vi "Read Serial Input Channel IO.vi"(0 "serial input channel io":T1, 2 "select corrected csi-2 data":bool) -> (4 "csi-2 data":u8[](array[numeric]), 6 "csi-2 status":T4, 10 "output valid":bool)   [LabVIEW 2020, in "GettingStarted_Acq_Tap_148X_FPGA.lvlib"]
uses:
  GettingStarted_Acq_Tap_148X_FPGA.lvlib
  Types/CSI-2 Status.ctl
  Types/Serial Input Channel IO.ctl
  Types/Serial Input Channel IO 32b.ctl
  Types/Serial Input Channel IO 64b.ctl
  <vilib>/rvi/eio/common/nirviEmuTemplateMethod_errors.vi
  <vilib>/eio/EIONode/EIONode.xnode
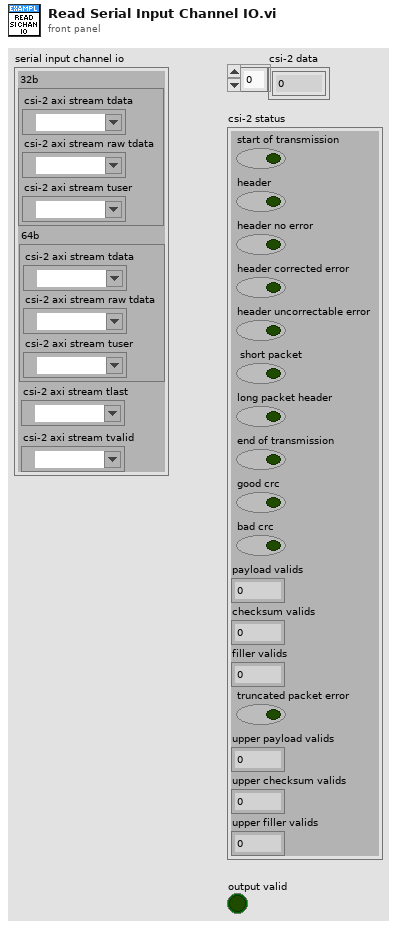
[diagram p1: front panel]
types:
  T1 = typedef "GettingStarted_Acq_Tap_148X_FPGA.lvlib/Serial Input Channel IO.ctl" = cluster{"32b":T2, "64b":T3, "csi-2 axi stream tlast":refnum<k21>, "csi-2 axi stream tvalid":refnum<k21>}
  T2 = typedef "GettingStarted_Acq_Tap_148X_FPGA.lvlib/Serial Input Channel IO 32b.ctl" = cluster{"csi-2 axi stream tdata":refnum<k21>, "csi-2 axi stream raw tdata":refnum<k21>, "csi-2 axi stream tuser":refnum<k21>}
  T3 = typedef "GettingStarted_Acq_Tap_148X_FPGA.lvlib/Serial Input Channel IO 64b.ctl" = cluster{"csi-2 axi stream tdata":refnum<k21>, "csi-2 axi stream raw tdata":refnum<k21>, "csi-2 axi stream tuser":refnum<k21>}
  T4 = typedef "GettingStarted_Acq_Tap_148X_FPGA.lvlib/CSI-2 Status.ctl" = cluster{"start of transmission":bool, "header":bool, "header no error":bool, "header corrected error":bool, "header uncorrectable error":bool, " short packet":bool, "long packet header":bool, "end of transmission":bool, "good crc":bool, "bad crc":bool, "payload valids":fxp<+,4,4>, "checksum valids":fxp<+,4,4>, "filler valids":fxp<+,4,4>, "truncated packet error":bool, "upper payload valids":fxp<+,4,4>, "upper checksum valids":fxp<+,4,4>, "upper filler valids":fxp<+,4,4>}
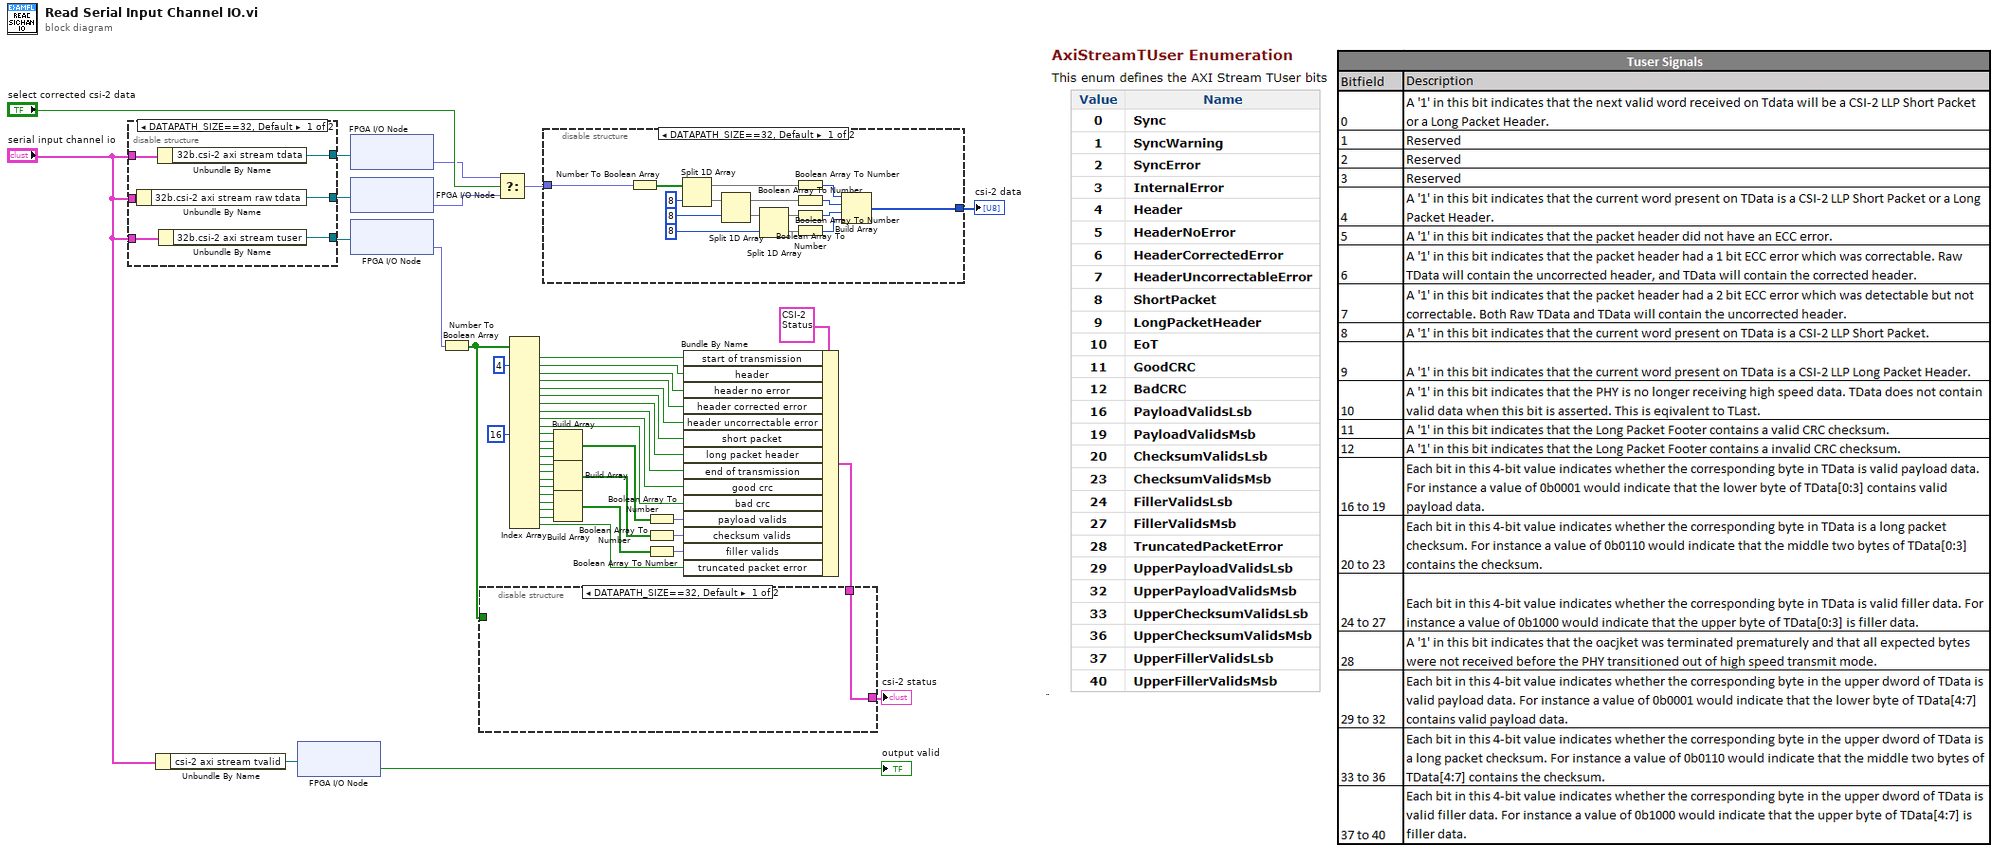
[diagram p0: block diagram]
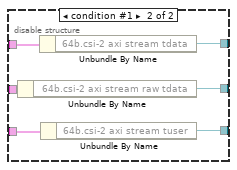
[diagram p2: hidden frame]
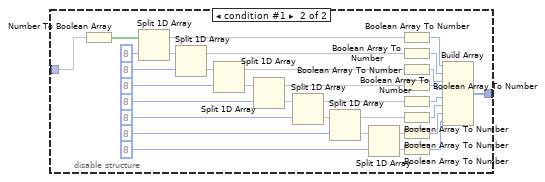
[diagram p3: hidden frame]
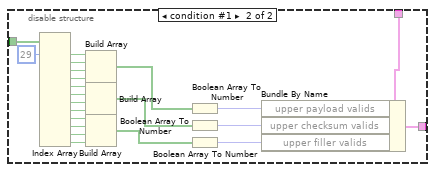
[diagram p4: hidden frame]
diagram:
  n1 = disable-structure shown="DATAPATH_SIZE==32, Default" {
    disable-tunnel: "serial input channel io" -> [w51 w59]
    disable-tunnel: "serial input channel io" -> [w52 w58]
    disable-tunnel: "serial input channel io" -> [w53 w57]
    disable-tunnel: [w50 w56] -> w6
    disable-tunnel: [w49 w55] -> w5
    disable-tunnel: [w48 w54] -> w4
    frame condition #0 (active) {
      n2 = Unbundle By Name(w52) -> ("32b.csi-2 axi stream raw tdata"=w49:refnum<k21>)
      n3 = Unbundle By Name(w53) -> ("32b.csi-2 axi stream tdata"=w48:refnum<k21>)
      n4 = Unbundle By Name(w51) -> ("32b.csi-2 axi stream tuser"=w50:refnum<k21>)
    }
    frame condition #1 {
      n5 = Unbundle By Name(w58) -> ("64b.csi-2 axi stream raw tdata"=w55:refnum<k21>)
      n6 = Unbundle By Name(w57) -> ("64b.csi-2 axi stream tdata"=w54:refnum<k21>)
      n7 = Unbundle By Name(w59) -> ("64b.csi-2 axi stream tuser"=w56:refnum<k21>)
    }
  }
  n8 = Unbundle By Name("serial input channel io") -> ("csi-2 axi stream tvalid"=w47:refnum<k21>)
  n9 = xnode "FPGA I/O Node"("FPGA I/O In"=w47) -> ("I/O Item"=→"output valid":bool)  [unwired: 1 out]
  n10 = xnode "FPGA I/O Node"("FPGA I/O In"=w4) -> ("I/O Item"=w42:fxp<+,32,32>)  [unwired: 1 out]
  n11 = xnode "FPGA I/O Node"("FPGA I/O In"=w5) -> ("I/O Item"=w41:fxp<+,32,32>)  [unwired: 1 out]
  n12 = xnode "FPGA I/O Node"("FPGA I/O In"=w6) -> ("I/O Item"=w45:fxp<+,32,32>)  [unwired: 1 out]
  n13 = Number To Boolean Array(number=w45) -> (Boolean array=w10:bool[])
  n14 = Select(t=w42, s="select corrected csi-2 data", f=w41) -> (s? t:f=w3:fxp<+,32,32>)
  n15 = Index Array(array=w10, index #2=4 ("index"), index #11=16 ("index")) -> (element #1=w46:bool, element #2=w38:bool, element #3=w37:bool, element #4=w36:bool, element #5=w35:bool, element #6=w34:bool, element #7=w33:bool, element #8=w32:bool, element #9=w31:bool, element #10=w30:bool, element #11=w28:bool, element #12=w27:bool, element #13=w26:bool, element #14=w25:bool, element #15=w23:bool, element #16=w22:bool, element #17=w21:bool, element #18=w20:bool, element #19=w17:bool, element #20=w16:bool, element #21=w15:bool, element #22=w14:bool, element #23=w1:bool)  [unwired: 21 in]
  n16 = disable-structure shown="DATAPATH_SIZE==32, Default" {
    disable-tunnel: w3 -> [w64 w94]
    disable-tunnel: [w60 w76] -> w2
    frame condition #0 (active) {
      n17 = Number To Boolean Array(number=w64) -> (Boolean array=w75:bool[])
      n18 = Split 1D Array(array=w75, index=8) -> (first subarray=w71:bool[], second subarray=w74:bool[])
      n19 = Split 1D Array(array=w74, index=8) -> (first subarray=w69:bool[], second subarray=w73:bool[])
      n20 = Split 1D Array(array=w73, index=8) -> (first subarray=w68:bool[], second subarray=w67:bool[])
      n21 = Boolean Array To Number(Boolean array=w71) -> (number=w72:u8)
      n22 = Boolean Array To Number(Boolean array=w69) -> (number=w70:u8)
      n23 = Boolean Array To Number(Boolean array=w68) -> (number=w66:u8)
      n24 = Boolean Array To Number(Boolean array=w67) -> (number=w65:u8)
      n25 = Build Array(w72, w70, w66, w65) -> (w60:u8[])
    }
    frame condition #1 {
      n26 = Number To Boolean Array(number=w94) -> (Boolean array=w107:bool[])
      n27 = Split 1D Array(array=w107, index=8) -> (first subarray=w103:bool[], second subarray=w106:bool[])
      n28 = Split 1D Array(array=w106, index=8) -> (first subarray=w101:bool[], second subarray=w105:bool[])
      n29 = Split 1D Array(array=w105, index=8) -> (first subarray=w100:bool[], second subarray=w93:bool[])
      n30 = Split 1D Array(array=w93, index=8) -> (first subarray=w92:bool[], second subarray=w91:bool[])
      n31 = Split 1D Array(array=w91, index=8) -> (first subarray=w90:bool[], second subarray=w89:bool[])
      n32 = Split 1D Array(array=w89, index=8) -> (first subarray=w88:bool[], second subarray=w87:bool[])
      n33 = Split 1D Array(array=w87, index=8) -> (first subarray=w86:bool[], second subarray=w85:bool[])
      n34 = Boolean Array To Number(Boolean array=w103) -> (number=w104:u8)
      n35 = Boolean Array To Number(Boolean array=w101) -> (number=w102:u8)
      n36 = Boolean Array To Number(Boolean array=w100) -> (number=w99:u8)
      n37 = Boolean Array To Number(Boolean array=w92) -> (number=w98:u8)
      n38 = Boolean Array To Number(Boolean array=w90) -> (number=w80:u8)
      n39 = Boolean Array To Number(Boolean array=w88) -> (number=w79:u8)
      n40 = Boolean Array To Number(Boolean array=w86) -> (number=w78:u8)
      n41 = Boolean Array To Number(Boolean array=w85) -> (number=w77:u8)
      n42 = Build Array(w104, w102, w99, w98, w80, w79, w78, w77) -> (w76:u8[])
    }
  }
  "csi-2 data" <- w2
  n43 = Build Array(w28, w27, w26, w25) -> (w24:bool[])
  n44 = Build Array(w23, w22, w21, w20) -> (w18:bool[])
  n45 = Build Array(w17, w16, w15, w14) -> (w12:bool[])
  n46 = Boolean Array To Number(Boolean array=w24) -> (number=w29:fxp<+,4,4>)
  n47 = Boolean Array To Number(Boolean array=w18) -> (number=w19:fxp<+,4,4>)
  n48 = Boolean Array To Number(Boolean array=w12) -> (number=w13:fxp<+,4,4>)
  n49 = Bundle By Name(cluster=T4 {"start of transmission"=FALSE, "header"=FALSE, "header no error"=FALSE, "header corrected error"=FALSE, "header uncorrectable error"=FALSE, " short packet"=FALSE, "long packet header"=FALSE, "end of transmission"=FALSE, "good crc"=FALSE, "bad crc"=FALSE, "payload valids"=0.0, "checksum valids"=0.0, "filler valids"=0.0, "truncated packet error"=FALSE, "upper payload valids"=0.0, "upper checksum valids"=0.0, "upper filler valids"=0.0}, "start of transmission"=w46, "header"=w38, "header no error"=w37, "header corrected error"=w36, "header uncorrectable error"=w35, "short packet"=w34, "long packet header"=w33, "end of transmission"=w32, "good crc"=w31, "bad crc"=w30, "payload valids"=w29, "checksum valids"=w19, "filler valids"=w13, "truncated packet error"=w1) -> (w9:T4)
  n50 = disable-structure shown="DATAPATH_SIZE==32, Default" {
    disable-tunnel: w10 -> [_ w126]
    disable-tunnel: w9 -> [w108 w110]
    disable-tunnel: [w108 w109] -> w8
    frame condition #0 (active) {
    }
    frame condition #1 {
      n51 = Index Array(array=w126, index #1=29 ("index")) -> (element #1=w127:bool, element #2=w125:bool, element #3=w124:bool, element #4=w123:bool, element #5=w122:bool, element #6=w121:bool, element #7=w120:bool, element #8=w119:bool, element #9=w118:bool, element #10=w117:bool, element #11=w116:bool, element #12=w115:bool)  [unwired: 11 in]
      n52 = Build Array(w127, w125, w124, w123) -> (w114:bool[])
      n53 = Build Array(w122, w121, w120, w119) -> (w129:bool[])
      n54 = Build Array(w118, w117, w116, w115) -> (w128:bool[])
      n55 = Boolean Array To Number(Boolean array=w114) -> (number=w113:fxp<+,4,4>)
      n56 = Boolean Array To Number(Boolean array=w129) -> (number=w112:fxp<+,4,4>)
      n57 = Boolean Array To Number(Boolean array=w128) -> (number=w111:fxp<+,4,4>)
      n58 = Bundle By Name(cluster=w110, "upper payload valids"=w113, "upper checksum valids"=w112, "upper filler valids"=w111) -> (w109:T4)
    }
  }
  "csi-2 status" <- w8
